vi "usrp get tx gain.vi"(7 "gain_out":dbl, 8 "error in (no error)":errorcluster, 9 "gain_name":string, 10 "chan":u64, 11 "h":u64) -> (0 "error out":errorcluster, 2 "function return":u32(ring), 3 "h 2":u64, 5 "gain_out out":dbl)   [LabVIEW 2024, in "uhd.lvlib"]
doc: "UHD_API uhd_error uhd_usrp_get_tx_gain(\n uhd_usrp_handle h, size_t chan, const char* gain_name, double* gain_out);"
uses:
  uhd.lvlib
  uhd.so
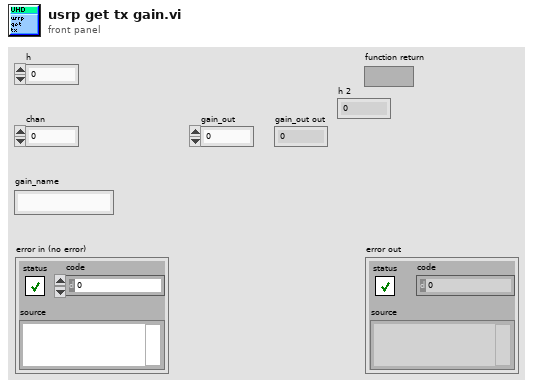
[diagram p1: front panel]
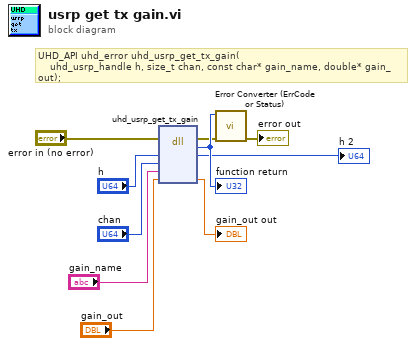
[diagram p0: block diagram]
diagram:
  # "UHD_API uhd_error uhd_usrp_get_tx_gain(\n    uhd_usrp_handle h, size_t chan, const char* gain_name, double* gain_out);"
  n1 = dll-call lib="uhd.*" fn="uhd_usrp_get_tx_gain"(error in="error in (no error)", "h"="h", "chan"="chan", "gain_name"="gain_name", "gain_out"="gain_out") -> (error out=w3:errorcluster, w10:u32, "h"=→"h 2":u64, "gain_out"=→"gain_out out":dbl)  [unwired: 4 in, 1 out]
  "function return" <- w10
  n2 = call "Error Converter (ErrCode or Status).vi"("error in (no error)"=w3, "error code"=w10) -> ("error out"=→"error out":errorcluster)  [unwired: 9 in]
